vi "ex_createNewChannelsTDM.vi"(0 "DAQmx Task":T1, 5 "signals":waveform(dbl)[](array[waveform]), 7 "file params":T6 {"Flags"."time preference" items=["Absolute", "Relative"]; "Flags"."x_columns" items=["None", "One", "Multiple"]; "origin time" format="%<%X\n%x>T"}, 9 "File path":path, 11 "error in (no error)":errorcluster, 12 "Comment":string, 13 "Description":string, 14 "write file properties":bool, 15 "append info in":T5) -> (4 "append info out":T5, 6 "bytes written":i32, 8 "error out":errorcluster)   [LabVIEW 2020]
uses:
  storage/Storage.llb/__savePropString.vi
  storage/lvStorage.llb/_wf_attributes.ctl
  storage/lvStorage.llb/_stringsToBeTranslated.ctl
  storage/Storage.llb/__savePropFloat64.vi
  express/express input/ExFileReadBlock.llb/ex_ReadFileParams.ctl
  express/express output/ExFileWriteBlock.llb/ex_WriteFileParams.ctl
  ex_appendInfoTDM.ctl
  express/express shared/ex_EditUserDefinedProperties/usiDataType.ctl
  express/express shared/ExFile.llb/ex_propertySource.ctl
  express/express shared/ExFile.llb/ex_userDefProperty.ctl
  express/express shared/ex_EditUserDefinedProperties/ex_userdefproperties.ctl
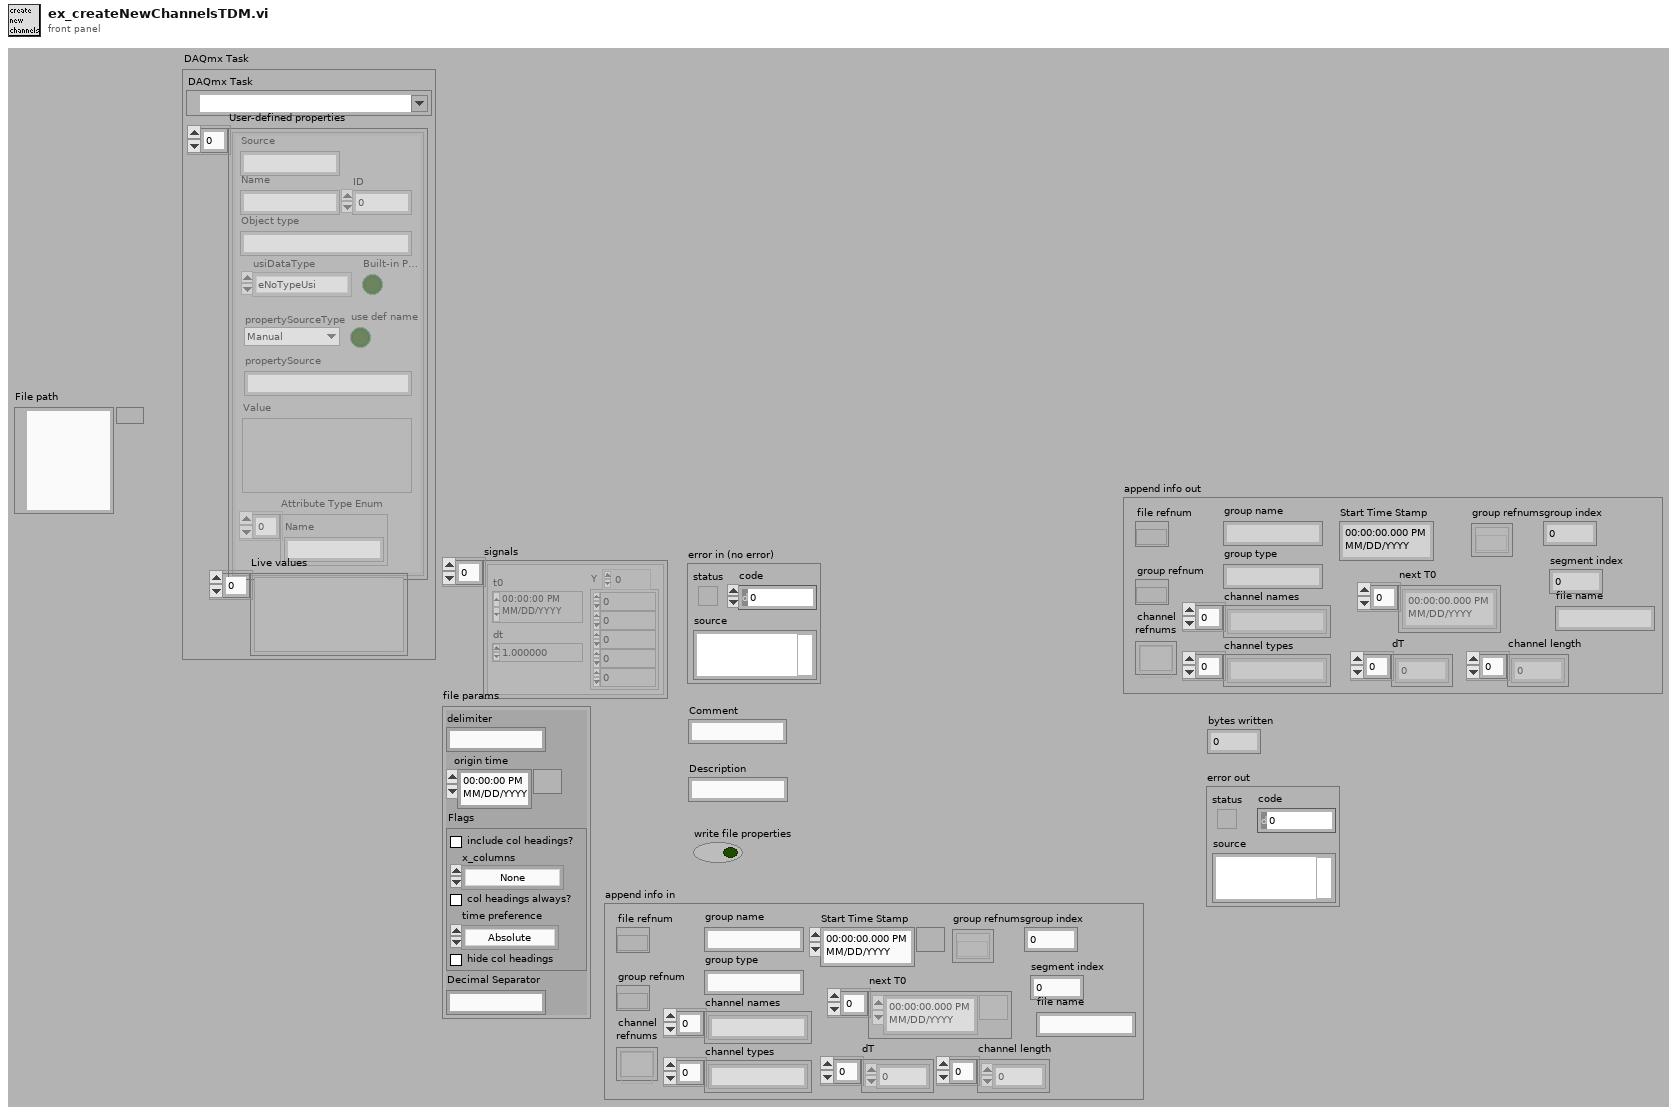
[diagram p1: front panel]
types:
  T1 = typedef "ex_userdefproperties.ctl" = cluster{"DAQmx Task":refnum<k21>, "User-defined properties":T2[], "Live values":variant[]}
  T2 = typedef "ex_userDefProperty.ctl" = cluster{"Name":string, "Object type":string, "usiDataType":T3, "propertySourceType":T4, "propertySource":string, "Value":variant, "ID":i32, "use def name":bool, "Source":string, "Built-in Prop":bool, "Attribute Type Enum":string[]}
  T3 = typedef "usiDataType.ctl" = enum16{"eNoTypeUsi", "eInt8Usi", "eInt16Usi", "eInt32Usi", "eInt64Usi", "eUInt8Usi", "eUInt16Usi", "eUInt32Usi", "eUInt64Usi", "eFloat32Usi", "eFloat64Usi", "- 0", "- 1", "- 2", "- 3", "- 4", "- 5", "- 6", "- 7", "- 8", "- 9", "eString8Usi", "eString16Usi", "eStringUsi", "eEnumUsi", "- 10", "- 11", "- 12", "- 13", "- 14", "eTimeUsi", "- 15", "- 16", "- 17", "- 18", "- 19", "- 20", "- 21", "- 22", "- 23", "eInstanceUsi", "eStoreUsi"}
  T4 = typedef "ex_propertySource.ctl" = enum16{"Manual", "System", "DAQmx Channel", "Terminal", "Ignore"}
  T5 = typedef "ex_appendInfoTDM.ctl" = cluster{"channel\nrefnums":refnum<k20>[], "channel names":string[], "channel types":string[], "file refnum":refnum<k20>, "group refnum":refnum<k20>, "group name":string, "group type":string, "next T0":timestamp[], "dT":dbl[], "Start Time Stamp":timestamp, "channel length":u32[], "group index":u32, "group refnums":refnum<k20>[], "file name":string, "segment index":u32}
  T6 = typedef "ex_WriteFileParams.ctl" = cluster{"delimiter":string, "origin time":timestamp, "Flags":T7, "Decimal Separator":string}
  T7 = typedef "ex_ReadFileParams.ctl" = cluster{"include col headings?":bool, "x_columns":u16, "col headings always?":bool, "time preference":u16, "hide col headings":bool}
  T8 = typedef "_stringsToBeTranslated.ctl" = enum16{"Properties", "View as icon", "query all data", "Load Storage VI parameters into memory", "Dynamically assign format", "Enumerated type", "Time stamp", "Configure", "Size to text", "Untitled", "storage refnum", "Load waveform data", "TDM (...)", "LVM (...)", "CSV (...)", "DYN (...)", "WrittenByLabVIEW", "TDMS", "out"}
  T9 = typedef "_wf_attributes.ctl" = enum16{"t0", "dt", "X_Name", "X_Unit", "x0", "abs/rel", "nPoints", "file_timestamp", "xcolumns"}
  T10 = typedef "ex_TdmData.ctl" = cluster{"New file":bool, "New header":bool, "File properties":T11[], "Header properties":T11[], "Signal properties":T11[][], "Signal values":waveform(dbl)[]}
  T11 = typedef "ex_TdmProperty.ctl" = cluster{"Name":string, "Type":T3, "Value":variant}
  T12 = cluster{"Start Timestamp":timestamp, "Timestamp":timestamp, "Relative Time?":bool, "X Dimension":string, "Signal Name":string, "Y Units":string, "X0":timestamp, "dX":dbl, "nPoints":i32}[]
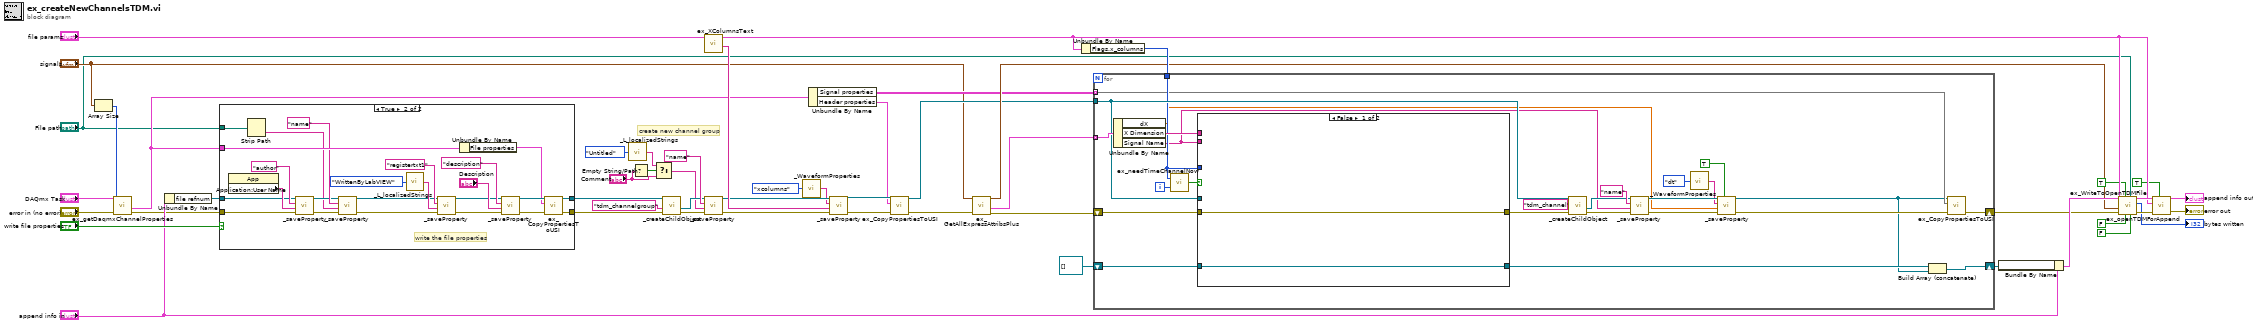
[diagram p0: block diagram]
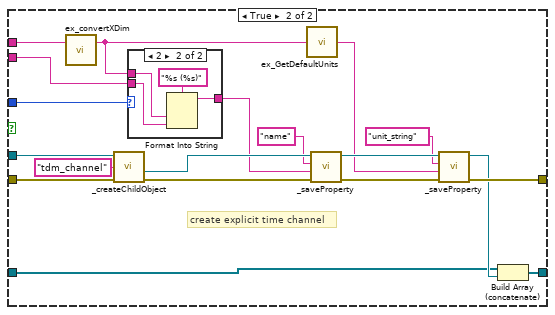
[diagram p3: hidden frame]
diagram:
  # "create new channel group"
  n1 = Array Size(array="signals") -> (size(s)=w8:i32)
  n2 = call "ex_getDaqmxChannelProperties.vi"("error in (no error)"="error in (no error)", "Number of channels (if no DAQmx task available)"=w8, "task"="DAQmx Task") -> ("error out"=w18:errorcluster, "all properties"=w12:T10)  [unwired: 1 in, 2 out]
  n3 = Unbundle By Name("append info in") -> ("file refnum"=w47:refnum<k20>)
  n4 = case shown="True" "write file properties" {
    tunnel: [w52 w69] -> w48
    tunnel: [w53 w68] -> w46
    tunnel: w47 -> [w53 w73]
    tunnel: w18 -> [w52 w72]
    tunnel: w12 -> [_ w67]
    tunnel: "File path" -> [_ w63]
    frame False {
      # "don't write file properties"
    }
    frame True {
      # "write the file properties"
      n5 = property class="App"() -> ("Application:User Name"=w75:string)  [unwired: 2 in, 2 out]
      n6 = Strip Path(path=w63) -> (name=w62:string)  [unwired: 1 out]
      n7 = call-poly "_saveProperty.vi"("error in (no error)"=w72, "Value"=w75, "Property name"="author", "storage refnum"=w73) -> ("error out"=w65:errorcluster, "dup storage refnum"=w64:refnum<k20>)  [unwired: 1 in, 5 out]
      n8 = call-poly "_saveProperty.vi"("error in (no error)"=w65, "Value"=w62, "Property name"="name", "storage refnum"=w64) -> ("error out"=w58:errorcluster, "dup storage refnum"=w57:refnum<k20>)  [unwired: 1 in, 5 out]
      n9 = call "_L_localizedStrings.vi"(1:_stringsToBeTranslated."WrittenByLabVIEW") -> (0:w61:string)
      n10 = call-poly "_saveProperty.vi"("error in (no error)"=w58, "Value"=w61, "Property name"="registertxt1", "storage refnum"=w57) -> ("error out"=w55:errorcluster, "dup storage refnum"=w56:refnum<k20>)  [unwired: 1 in, 5 out]
      n11 = Unbundle By Name(w67) -> ("File properties"=w54:T11[])
      n12 = call-poly "_saveProperty.vi"("error in (no error)"=w55, "Value"="Description", "Property name"="description", "storage refnum"=w56) -> ("error out"=w70:errorcluster, "dup storage refnum"=w71:refnum<k20>)  [unwired: 1 in, 5 out]
      n13 = call "ex_CopyPropertiesToUSI.vi"("error in (no error)"=w70, "Properties"=w54, "dup storage refnum"=w71) -> ("error out"=w69:errorcluster, "dup storage refnum"=w68:refnum<k20>)  [unwired: 1 in, 2 out]
    }
  }
  n14 = call "_L_localizedStrings.vi"(1:_stringsToBeTranslated."Untitled") -> (0:w7:string)
  n15 = Empty String/Path?(string/path="Comment") -> (empty?=w5:bool)
  n16 = Select(t=w7, s=w5, f="Comment") -> (s? t:f=w3:string)
  n17 = call "_createChildObject.vi"("error in (no error)"=w48, "Object type"="tdm_channelgroup", "storage refnum"=w46) -> ("error out"=w31:errorcluster, "new storage refnum"=w33:refnum<k20>)  [unwired: 3 out]
  n18 = call "ex_XColumnsText.vi"("file info in"="file params") -> ("xcolumns"=w50:string, "file info out"=w41:T6)  [unwired: 5 out]
  n19 = call-poly "_saveProperty.vi"("error in (no error)"=w31, "Value"=w3, "Property name"="name", "storage refnum"=w33) -> ("error out"=w30:errorcluster, "dup storage refnum"=w29:refnum<k20>)  [unwired: 1 in, 5 out]
  n20 = call "_WaveformProperties.vi"("Property"=_wf_attributes."xcolumns") -> ("Name"=w28:string)
  n21 = Unbundle By Name(w12) -> ("Signal properties"=w11:T11[][], "Header properties"=w2:T11[])
  n22 = call-poly "_saveProperty.vi"("error in (no error)"=w30, "Value"=w50, "Property name"=w28, "storage refnum"=w29) -> ("error out"=w16:errorcluster, "dup storage refnum"=w14:refnum<k20>)  [unwired: 1 in, 5 out]
  n23 = call "ex_CopyPropertiesToUSI.vi"("error in (no error)"=w16, "Properties"=w2, "dup storage refnum"=w14) -> ("error out"=w15:errorcluster, "dup storage refnum"=w13:refnum<k20>)  [unwired: 1 in, 2 out]
  n24 = call "ex_GetAllExpressAttribsPlus.vi"("error in"=w15, "Signals in"="signals") -> ("error out"=w10:errorcluster, "All Express Wave Attributes Plus"=w26:T12, "Signals out"=w25:waveform(dbl)[])  [unwired: 7 out]
  n25 = Unbundle By Name(w41) -> ("Flags.x_columns"=w45:u16)
  n26 = for {
    tunnel: w26 -> [w102] mode=indexing
    shift-right: [w87] -> w21
    shift-left: w10 -> [w103]
    tunnel: w13 -> [w95]
    tunnel: w45 -> [w92]
    shift-right: [w89] -> w37
    shift-left: refnum<k20>[] [] -> [w88]
    tunnel: w11 -> [w86] mode=indexing
    i -> [w100]
    n27 = Unbundle By Name(w102) -> ("dX"=w79:dbl, "X Dimension"=w94:string, "Signal Name"=w91:string)
    n28 = call "ex_needTimeChannelNow.vi"("index"=w100, "x_columns"=w92) -> ("need time channel NOW !!!!"=w93:bool)
    n29 = case shown="False" w93 {
      tunnel: w95 -> [_ w124]
      tunnel: w103 -> [w105 w123]
      tunnel: [w105 w113] -> w98
      tunnel: w91 -> [_ w114]
      tunnel: w94 -> [_ w111]
      tunnel: w92 -> [_ w112]
      tunnel: [w104 w107] -> w90
      tunnel: w88 -> [w104 w106]
      frame False {
      }
      frame True {
        # "create explicit time channel"
        n30 = call "ex_convertXDim.vi"("x_dimension in"=w111) -> ("x_dimension out"=w110:string)  [unwired: 1 in, 1 out]
        n31 = call "_createChildObject.vi"("error in (no error)"=w123, "Object type"="tdm_channel", "storage refnum"=w124) -> ("error out"=w121:errorcluster, "new storage refnum"=w120:refnum<k20>)  [unwired: 2 in, 1 out]
        n32 = case shown="2" w112 {
          tunnel: [w125 w128] -> w118
          tunnel: w110 -> [w125 w127]
          tunnel: w114 -> [_ w126]
          frame Default {
          }
          frame 2 {
            n33 = Format Into String(format string="%s (%s)", w127, w126) -> (resulting string=w128:string)  [unwired: 2 in, 1 out]
          }
        }
        n34 = call "ex_GetDefaultUnits.vi"("dimension"=w110) -> ("default units"=w109:string)
        n35 = call-poly "_saveProperty.vi"("error in (no error)"=w121, "Value"=w118, "Property name"="name", "storage refnum"=w120) -> ("error out"=w117:errorcluster, "dup storage refnum"=w116:refnum<k20>)  [unwired: 1 in, 5 out]
        n36 = call-poly "_saveProperty.vi"("error in (no error)"=w117, "Value"=w109, "Property name"="unit_string", "storage refnum"=w116) -> ("error out"=w113:errorcluster, "dup storage refnum"=w108:refnum<k20>)  [unwired: 1 in, 5 out]
        n37 = Build Array (concatenate)(w106, w108) -> (w107:refnum<k20>[])
      }
    }
    n38 = call "_createChildObject.vi"("error in (no error)"=w98, "Object type"="tdm_channel", "storage refnum"=w95) -> ("error out"=w97:errorcluster, "new storage refnum"=w96:refnum<k20>)  [unwired: 2 in, 1 out]
    n39 = call-poly "_saveProperty.vi"("error in (no error)"=w97, "Value"=w91, "Property name"="name", "storage refnum"=w96) -> ("error out"=w84:errorcluster, "dup storage refnum"=w85:refnum<k20>)  [unwired: 1 in, 5 out]
    n40 = call "_WaveformProperties.vi"("Property"=_wf_attributes."dt") -> ("Name"=w80:string)
    n41 = call-poly "_saveProperty.vi"("User-defined property"=TRUE, "error in (no error)"=w84, "Value"=w79, "Property name"=w80, "storage refnum"=w85) -> ("error out"=w83:errorcluster, "dup storage refnum"=w82:refnum<k20>)  [unwired: 5 out]
    n42 = Build Array (concatenate)(w90, w82) -> (w89:refnum<k20>[])
    n43 = call "ex_CopyPropertiesToUSI.vi"("error in (no error)"=w83, "Properties"=w86, "dup storage refnum"=w82) -> ("error out"=w87:errorcluster)  [unwired: 1 in, 3 out]
  }
  n44 = Bundle By Name(cluster="append info in", "channel\nrefnums"=w37) -> (w39:T5)
  n45 = call "ex_WriteToOpenTDMFile.vi"("error if check fails"=FALSE, "File path in"="File path", "check time attributes"=FALSE, "write ddt attr"=TRUE, "error in (no error)"=w21, "Signals"=w25, "file params"=w41, "append info in"=w39) -> ("error out"=w42:errorcluster, "bytes written"=→"bytes written":i32, "append info out"=w43:T5)  [unwired: 1 out]
  n46 = call "ex_openTDMForAppend.vi"("always read cache"=TRUE, "error in (no error)"=w42, "file params"=w41, "append info in"=w43) -> ("error out"=→"error out":errorcluster, "append info out"=→"append info out":T5)  [unwired: 1 in, 5 out]
